vi "dispense test.vi"() -> ()   [LabVIEW 2020]
uses:
  Classes/Controller/Dispenser/Dispenser.lvclass
  Classes/Controller/Controller.lvclass
panel:
  out "std":dbl
  out "average":dbl
  out "Time":u32[](array[numeric])
  in  "N":i32
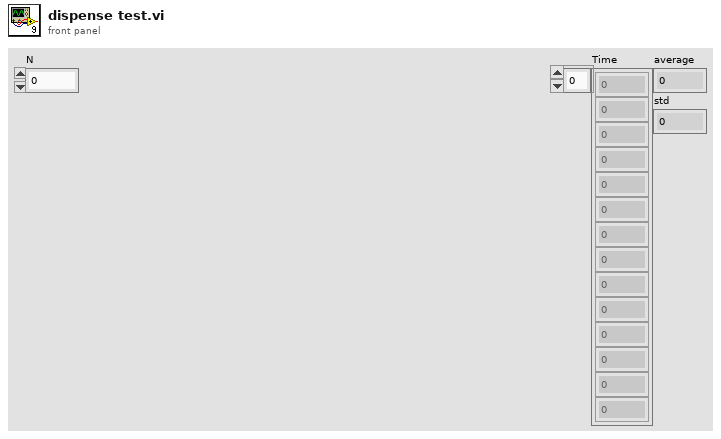
[diagram p1: front panel]
types:
  T1 = typedef "Controller.lvclass/Controllers.ctl" = cluster{"I-O.lvclass":refnum<class "I-O.lvclass">, "Dispenser.lvclass":refnum<class "Dispenser.lvclass">, "Gantry":refnum<k24>}
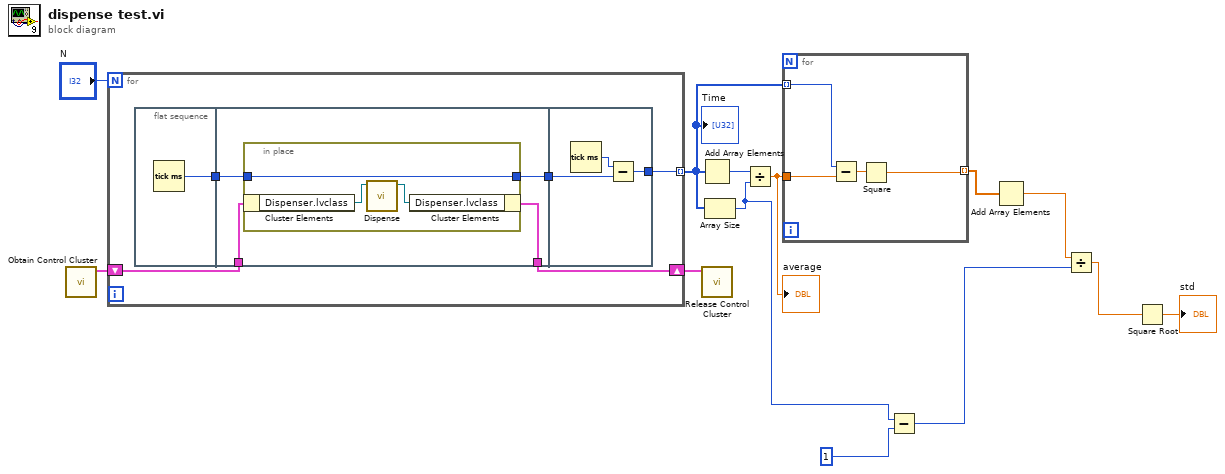
[diagram p0: block diagram]
diagram:
  n1 = call "Obtain Control Cluster.vi"() -> ("Control Out"=w13:T1)  [unwired: 11 in]
  n2 = for {
    N: "N" -> [_]
    tunnel: [w16] -> w9 mode=indexing
    shift-right: [w14] -> w12
    shift-left: w13 -> [w15]
    n3 = flat-sequence {
      tunnel: [w19] -> w18
      tunnel: w18 -> [w23]
      tunnel: [w22] -> w17
      tunnel: [w21] -> w14
      tunnel: w15 -> [w20]
      tunnel: w17 -> [w28]
      tunnel: [w27] -> w16
      frame #0 {
        n4 = Tick Count (ms)() -> (millisecond timer value=w19:u32)
      }
      frame #1 {
        n5 = in-place {
          in-place-border: w23 -> [w26]
          in-place-border: [w26] -> w22
          n6 = in-place-cluster #1(w20) -> ("Dispenser.lvclass"=w24:refnum<class "Dispenser.lvclass">)
          n7 = call-dynamic "Dispense.vi"("Dispenser in"=w24) -> ("Dispenser out"=w25:refnum<class "Dispenser.lvclass">)  [unwired: 9 in, 1 out]
          n8 = in-place-cluster #1("Dispenser.lvclass"=w25) -> (w21:T1)
        }
      }
      frame #2 {
        n9 = Tick Count (ms)() -> (millisecond timer value=w29:u32)
        n10 = Subtract(x=w29, y=w28) -> (x-y=w27:u32)
      }
    }
  }
  "Time" <- w9
  n11 = Add Array Elements(numeric array=w9) -> (sum=w10:u32)
  n12 = call "Release Control Cluster.vi"("output cluster"=w12) -> ()  [unwired: 11 in]
  n13 = Array Size(array=w9) -> (size(s)=w4:i32)
  n14 = Divide(x=w10, y=w4) -> (x/y=w8:dbl)
  "average" <- w8
  n15 = for {
    tunnel: w9 -> [w33] mode=indexing
    tunnel: w8 -> [w32]
    tunnel: [w30] -> w7 mode=indexing
    n16 = Subtract(x=w33, y=w32) -> (x-y=w31:dbl)
    n17 = Square(x=w31) -> (x^2=w30:dbl)
  }
  n18 = Subtract(x=w4, y=1) -> (x-y=w3:i32)
  n19 = Add Array Elements(numeric array=w7) -> (sum=w6:dbl)
  n20 = Divide(x=w6, y=w3) -> (x/y=w2:dbl)
  n21 = Square Root(x=w2) -> (sqrt(x)=→"std":dbl)
